vi "3-Enconders_2-Digital.vi"   [LabVIEW 2015]
uses:
  <vilib>/Rock Robotics/WPI/Encoder/WPI_EncoderType.ctl
  <vilib>/Rock Robotics/SystemInterfaces/DIO/FPGA_DIOChannel.ctl
  Global_Var/Drive_Global.vi
  <vilib>/Rock Robotics/WPI/Counter/WPI_CounterDigitalInputToDigitalSource.vi
  <vilib>/Rock Robotics/WPI/Counter/WPI_CounterOpen UpDown Mode.vi
  <vilib>/Rock Robotics/WPI/Ultrasonic/WPI_SonarMB1010DigitalOpen.vi
  <vilib>/Rock Robotics/WPI/Ultrasonic/WPI_SonarMB1010DigRefNum Registry Set.vi
panel:
  # "Created by Matt Carr on 1/25/2016"
types:
  T1 = typedef "WPI_EncoderType.ctl" = enum16{"1x", "2x", "4x"}
  T2 = typedef "FPGA_DIOChannel.ctl" = enum8{"DIO 0", "DIO 1", "DIO 2", "DIO 3", "DIO 4", "DIO 5", "DIO 6", "DIO 7", "DIO 8", "DIO 9", "DIO MXP 0", "DIO MXP 1", "DIO MXP 2", "DIO MXP 3", "DIO MXP 4", "DIO MXP 5", "DIO MXP 6", "DIO MXP 7", "DIO MXP 8", "DIO MXP 9", "DIO MXP 10", "DIO MXP 11", "DIO MXP 12", "DIO MXP 13", "DIO MXP 14", "DIO MXP 15", "Invalid"}
  T3 = typedef "WPI_DigitalInputDevRef.ctl" = cluster{"DevStatus":errorcluster, "DIO Channel":T2}
  T4 = typedef "WPI_SonarMB1010DigitalDeviceRef.ctl" = cluster{"CounterDevRef":T5, "Scaling factor (s/in)":dbl}
  T5 = typedef "WPI_CounterDevRef.ctl" = cluster{"DevStatus":errorcluster, "CntIndex":T6}
  T6 = typedef "FPGA_CounterCtrSystemIndex.ctl" = enum8{"Ctr 0", "Ctr 1", "Ctr 2", "Ctr 3", "Ctr 4", "Ctr 5", "Ctr 6", "Ctr 7", "Invalid"}
  T7 = typedef "FPGA_CounterEncoderSourceConvertionLVSourceType.ctl" = cluster{"DevStatus":errorcluster, "AnalogTriggerMode?":bool, "DigitalMode":cluster{"DIO Channel":T8}, "AnalogTriggerMode":cluster{"AnalogTriggerIndex":T9, "OutputType":T10}}
  T8 = typedef "FPGA_DIODigitalSourceChannel.ctl" = enum8{"DIO 0", "DIO 1", "DIO 2", "DIO 3", "DIO 4", "DIO 5", "DIO 6", "DIO 7", "DIO 8", "DIO 9", "DIO MXP 0", "DIO MXP 1", "DIO MXP 2", "DIO MXP 3", "DIO MXP 4", "DIO MXP 5", "DIO MXP 6", "DIO MXP 7", "DIO MXP 8", "DIO MXP 9", "DIO MXP 10", "DIO MXP 11", "DIO MXP 12", "DIO MXP 13", "DIO MXP 14", "DIO MXP 15", "Disabled"}
  T9 = typedef "FPGA_AnalogTriggerIndex.ctl" = enum8{"Trig 0", "Trig 1", "Trig 2", "Trig 3", "Trig 4", "Trig 5", "Trig 6", "Trig 7", "Invalid"}
  T10 = typedef "FPGA_AnalogTriggerOutType.ctl" = enum16{"InWindow", "TriggerState", "Rising", "Falling"}
  T11 = typedef "WPI_EncoderDevRef.ctl" = cluster{"DevStatus":errorcluster, "EncoderIndex":T12, "CounterIndex":T6, "DistancePerCount":dbl, "Decoding Type":T1}
  T12 = typedef "FPGA_EncoderIdx.ctl" = enum8{"Enc 0", "Enc 1", "Enc 2", "Enc 3", "Enc 4", "Enc 5", "Enc 6", "Enc 7", "Invalid"}
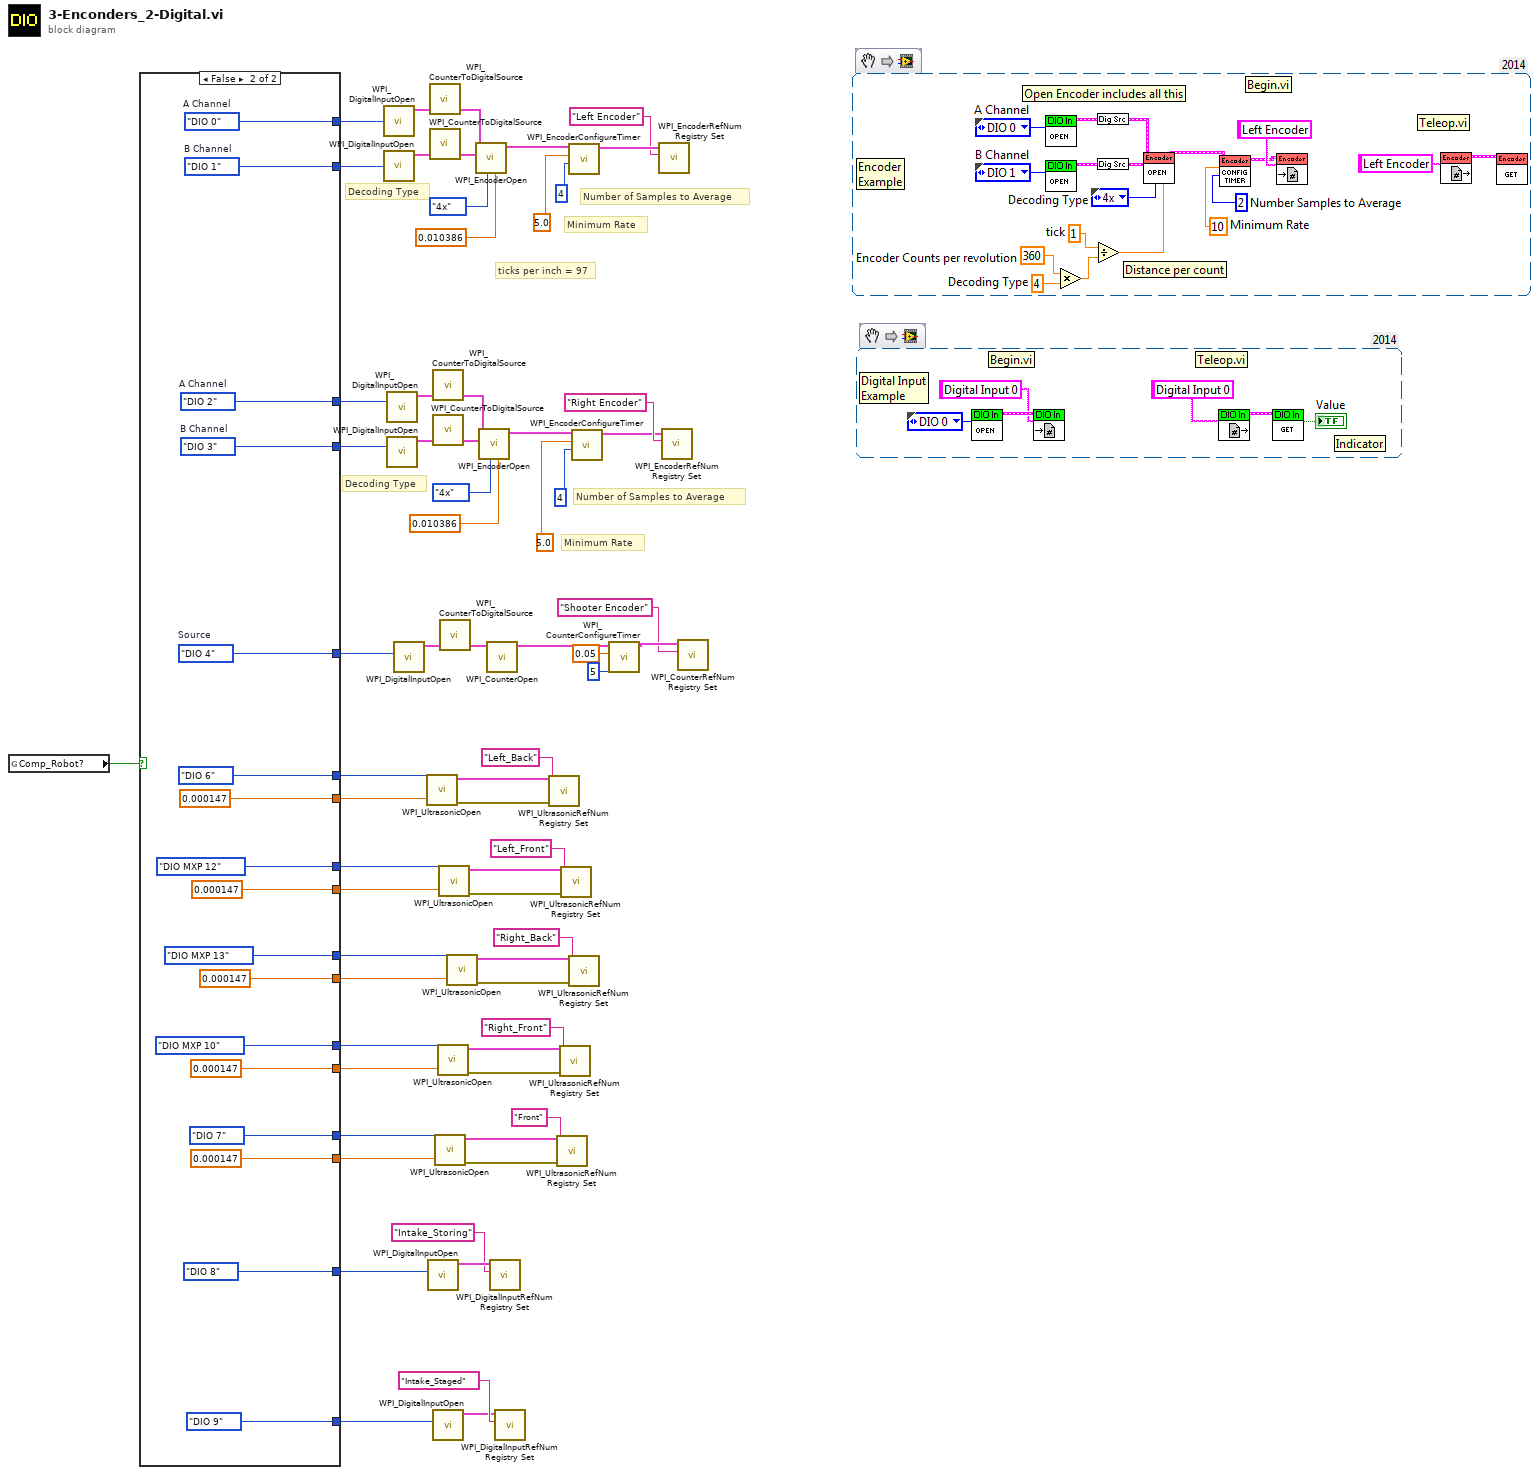
[diagram p0: block diagram]
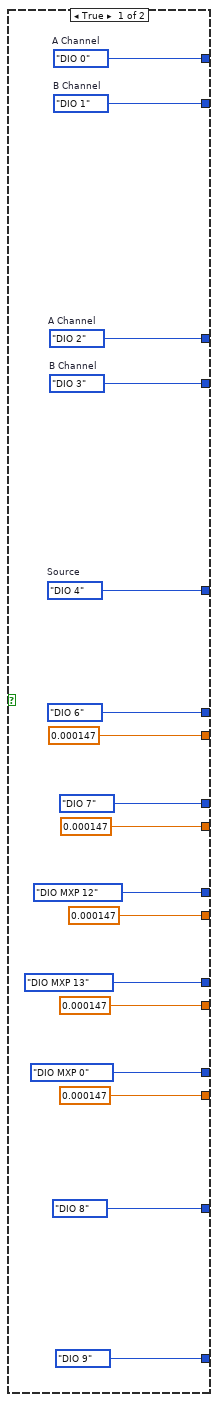
[diagram p2: hidden frame]
diagram:
  # "Decoding Type"
  # "Decoding Type"
  # "ticks per inch = 97"
  # "Number of Samples to Average"
  # "Minimum Rate"
  # "Minimum Rate"
  # "Number of Samples to Average"
  n1 = global read "Drive_Global.vi" "Comp_Robot?"() -> (w1:bool)
  n2 = case shown="False" w1 {
    tunnel: [w83 w100] -> w66
    tunnel: [w82 w99] -> w65
    tunnel: [w81 w98] -> w44
    tunnel: [w80 w97] -> w43
    tunnel: [FPGA_DIOChannel."DIO 8" ("DIO Channel") FPGA_DIOChannel."DIO 8" ("DIO Channel")] -> w42
    tunnel: [FPGA_DIOChannel."DIO 9" ("DIO Channel") FPGA_DIOChannel."DIO 9" ("DIO Channel")] -> w37
    tunnel: [FPGA_DIOChannel."DIO 6" ("DIO Channel") FPGA_DIOChannel."DIO 6" ("DIO Channel")] -> w36
    tunnel: [0.000147 ("Scaling factor (s/in)") 0.000147 ("Scaling factor (s/in)")] -> w35
    tunnel: [0.000147 ("Scaling factor (s/in)") 0.000147 ("Scaling factor (s/in)")] -> w28
    tunnel: [FPGA_DIOChannel."DIO 7" ("DIO Channel") FPGA_DIOChannel."DIO MXP 12" ("DIO Channel")] -> w27
    tunnel: [FPGA_DIOChannel."DIO MXP 12" ("DIO Channel") FPGA_DIOChannel."DIO MXP 13" ("DIO Channel")] -> w26
    tunnel: [0.000147 ("Scaling factor (s/in)") 0.000147 ("Scaling factor (s/in)")] -> w25
    tunnel: [0.000147 ("Scaling factor (s/in)") 0.000147 ("Scaling factor (s/in)")] -> w18
    tunnel: [FPGA_DIOChannel."DIO MXP 13" ("DIO Channel") FPGA_DIOChannel."DIO MXP 10" ("DIO Channel")] -> w17
    tunnel: [FPGA_DIOChannel."DIO MXP 0" ("DIO Channel") FPGA_DIOChannel."DIO 7" ("DIO Channel")] -> w16
    tunnel: [0.000147 ("Scaling factor (s/in)") 0.000147 ("Scaling factor (s/in)")] -> w15
    tunnel: [w67 w84] -> w8
    frame True {
      w67 = FPGA_DIOChannel."DIO 4"  # Source
      w80 = FPGA_DIOChannel."DIO 3"  # B Channel
      w81 = FPGA_DIOChannel."DIO 2"  # A Channel
      w83 = FPGA_DIOChannel."DIO 1"  # B Channel
      w82 = FPGA_DIOChannel."DIO 0"  # A Channel
    }
    frame False {
      w84 = FPGA_DIOChannel."DIO 4"  # Source
      w97 = FPGA_DIOChannel."DIO 3"  # B Channel
      w98 = FPGA_DIOChannel."DIO 2"  # A Channel
      w100 = FPGA_DIOChannel."DIO 1"  # B Channel
      w99 = FPGA_DIOChannel."DIO 0"  # A Channel
    }
  }
  n3 = call <vilib>:"WPI_DigitalInputOpen.vi"("DIO Channel"=w65) -> ("DigitalInputDevRef"=w62:T3)  [unwired: 1 in, 9 out]
  n4 = call <vilib>:"WPI_DigitalInputOpen.vi"("DIO Channel"=w66) -> ("DigitalInputDevRef"=w63:T3)  [unwired: 1 in, 9 out]
  n5 = call <vilib>:"WPI_DigitalInputOpen.vi"("DIO Channel"=w44) -> ("DigitalInputDevRef"=w47:T3)  [unwired: 1 in, 9 out]
  n6 = call <vilib>:"WPI_DigitalInputOpen.vi"("DIO Channel"=w43) -> ("DigitalInputDevRef"=w46:T3)  [unwired: 1 in, 9 out]
  n7 = call <vilib>:"WPI_DigitalInputOpen.vi"("DIO Channel"=w8) -> ("DigitalInputDevRef"=w7:T3)  [unwired: 1 in, 9 out]
  n8 = call-poly <vilib>:"WPI_UltrasonicOpen.vi"("Scaling factor (s/in)"=w35, "DIO Channel"=w36) -> ("error out"=w33:errorcluster, "SonarMB1010DigitalDevRef"=w34:T4)  [unwired: 8 in]
  n9 = call <vilib>:"WPI_DigitalInputOpen.vi"("DIO Channel"=w42) -> ("DigitalInputDevRef"=w41:T3)  [unwired: 9 in, 1 out]
  n10 = call-poly <vilib>:"WPI_CounterToDigitalSource.vi"("DigitalInputDevRef"=w62) -> ("Digital Source"=w61:T7)  [unwired: 6 out]
  n11 = call-poly <vilib>:"WPI_CounterToDigitalSource.vi"("DigitalInputDevRef"=w63) -> ("Digital Source"=w64:T7)  [unwired: 6 out]
  n12 = call-poly <vilib>:"WPI_CounterToDigitalSource.vi"("DigitalInputDevRef"=w47) -> ("Digital Source"=w48:T7)  [unwired: 6 out]
  n13 = call-poly <vilib>:"WPI_CounterToDigitalSource.vi"("DigitalInputDevRef"=w46) -> ("Digital Source"=w45:T7)  [unwired: 6 out]
  n14 = call <vilib>:"WPI_DigitalInputOpen.vi"("DIO Channel"=w37) -> ("DigitalInputDevRef"=w38:T3)  [unwired: 9 in, 1 out]
  n15 = call-poly <vilib>:"WPI_UltrasonicOpen.vi"("Scaling factor (s/in)"=w15, "DIO Channel"=w16) -> ("error out"=w13:errorcluster, "SonarMB1010DigitalDevRef"=w14:T4)  [unwired: 8 in]
  n16 = call-poly <vilib>:"WPI_UltrasonicOpen.vi"("Scaling factor (s/in)"=w18, "DIO Channel"=w17) -> ("error out"=w20:errorcluster, "SonarMB1010DigitalDevRef"=w19:T4)  [unwired: 8 in]
  n17 = call-poly <vilib>:"WPI_UltrasonicOpen.vi"("Scaling factor (s/in)"=w28, "DIO Channel"=w27) -> ("error out"=w30:errorcluster, "SonarMB1010DigitalDevRef"=w29:T4)  [unwired: 8 in]
  n18 = call-poly <vilib>:"WPI_CounterToDigitalSource.vi"("DigitalInputDevRef"=w7) -> ("Digital Source"=w9:T7)  [unwired: 6 out]
  n19 = call-poly <vilib>:"WPI_UltrasonicOpen.vi"("Scaling factor (s/in)"=w25, "DIO Channel"=w26) -> ("error out"=w23:errorcluster, "SonarMB1010DigitalDevRef"=w24:T4)  [unwired: 8 in]
  n20 = call <vilib>:"WPI_EncoderOpen.vi"("DistancePerCount"=0.010386, "Decoding Type"=WPI_EncoderType."4x", "BSource"=w64, "ASource"=w61) -> ("EncoderDevRef"=w59:T11)  [unwired: 4 in, 3 out]
  n21 = call <vilib>:"WPI_EncoderOpen.vi"("DistancePerCount"=0.010386, "Decoding Type"=WPI_EncoderType."4x", "BSource"=w45, "ASource"=w48) -> ("EncoderDevRef"=w50:T11)  [unwired: 4 in, 3 out]
  n22 = call-poly <vilib>:"WPI_CounterOpen.vi"("Up Source"=w9) -> ("CounterDevRef"=w6:T5)  [unwired: 6 in, 4 out]
  n23 = call <vilib>:"WPI_DigitalInputRefNum Registry Set.vi"("refnum name"="Intake_Storing", "DigitalInputDevRef"=w41) -> ()  [unwired: 8 in, 2 out]
  n24 = call <vilib>:"WPI_DigitalInputRefNum Registry Set.vi"("refnum name"="Intake_Staged", "DigitalInputDevRef"=w38) -> ()  [unwired: 8 in, 2 out]
  n25 = call-poly <vilib>:"WPI_UltrasonicRefNum Registry Set.vi"("error in (no error)"=w33, "refnum name"="Left_Back", "SonarMB1010DigitalDevRef"=w34) -> ()  [unwired: 7 in, 2 out]
  n26 = call-poly <vilib>:"WPI_UltrasonicRefNum Registry Set.vi"("error in (no error)"=w13, "refnum name"="Front", "SonarMB1010DigitalDevRef"=w14) -> ()  [unwired: 7 in, 2 out]
  n27 = call-poly <vilib>:"WPI_UltrasonicRefNum Registry Set.vi"("error in (no error)"=w20, "refnum name"="Right_Front", "SonarMB1010DigitalDevRef"=w19) -> ()  [unwired: 7 in, 2 out]
  n28 = call-poly <vilib>:"WPI_UltrasonicRefNum Registry Set.vi"("error in (no error)"=w30, "refnum name"="Left_Front", "SonarMB1010DigitalDevRef"=w29) -> ()  [unwired: 7 in, 2 out]
  n29 = call <vilib>:"WPI_EncoderConfigureTimer.vi"("Number Samples to Average"=u8 4, "Minimum Rate"=5.0, "EncoderDevRef"=w59) -> ("EncoderDevRef"=w56:T11)  [unwired: 7 in, 1 out]
  n30 = call-poly <vilib>:"WPI_UltrasonicRefNum Registry Set.vi"("error in (no error)"=w23, "refnum name"="Right_Back", "SonarMB1010DigitalDevRef"=w24) -> ()  [unwired: 7 in, 2 out]
  n31 = call <vilib>:"WPI_EncoderConfigureTimer.vi"("Number Samples to Average"=u8 4, "Minimum Rate"=5.0, "EncoderDevRef"=w50) -> ("EncoderDevRef"=w53:T11)  [unwired: 7 in, 1 out]
  n32 = call <vilib>:"WPI_CounterConfigureTimer.vi"("Number Samples to Average"=u8 5, "MaxPeriod (sec)"=0.05, "CounterDevRef in"=w6) -> ("CounterDevRef out"=w3:T5)  [unwired: 7 in, 1 out]
  n33 = call <vilib>:"WPI_EncoderRefNum Registry Set.vi"("refnum name"="Left Encoder", "EncoderDevRef"=w56) -> ()  [unwired: 8 in, 2 out]
  n34 = call <vilib>:"WPI_EncoderRefNum Registry Set.vi"("refnum name"="Right Encoder", "EncoderDevRef"=w53) -> ()  [unwired: 8 in, 2 out]
  n35 = call <vilib>:"WPI_CounterRefNum Registry Set.vi"("refnum name"="Shooter Encoder", "CounterDevRef"=w3) -> ()  [unwired: 8 in, 2 out]
